vi "movetowl.vi"(8 "error out":errorcluster, 9 "GetDeviceInterface":refnum<k7>, 10 "Wavelength":dbl=795.0) -> (2 ".not. (x .or. y)?":bool)   [LabVIEW 2019]
panel:
  out "Angle":dbl
  out "Wavelength 2":dbl
  out "Serial number":string
  out "Temperature":dbl
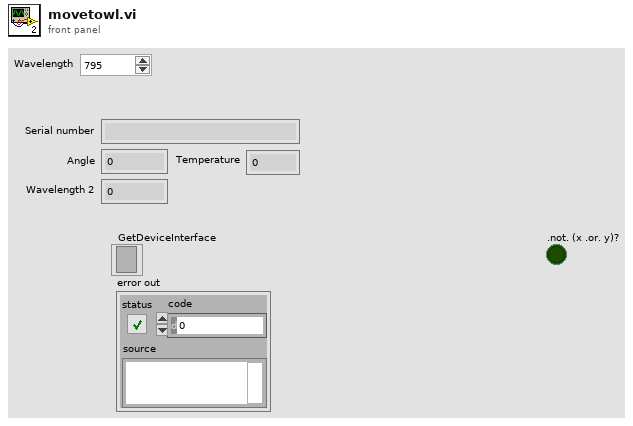
[diagram p1: front panel]
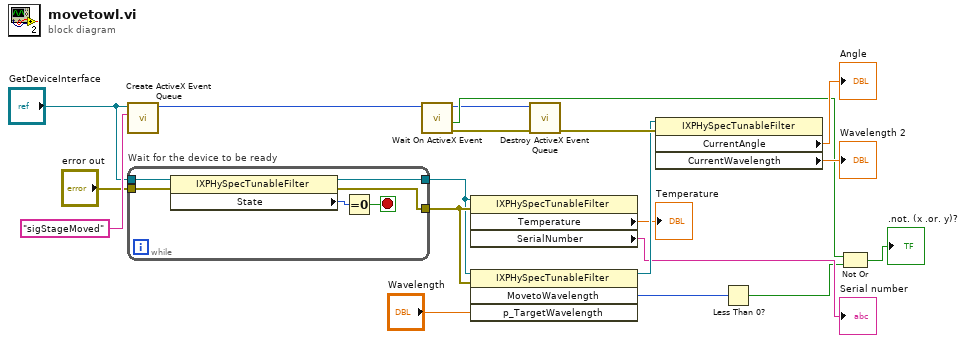
[diagram p0: block diagram]
diagram:
  n1 = call <vilib>:"Create ActiveX Event Queue.vi"("Event Name"="sigStageMoved", "Automation Refnum"="GetDeviceInterface") -> ("Event Queue"=w7:i32)  [unwired: 4 in, 1 out]
  n2 = while "Wait for the device to be ready" {
    tunnel: [w23] -> w5
    tunnel: "GetDeviceInterface" -> [w22]
    tunnel: "error out" -> [w21]
    tunnel: [w20] -> w4
    stop <- w24 stop-if-true
    n3 = property class="IXPHySpecTunableFilter"(reference=w22, error in=w21) -> (reference out=w20:refnum<k7>, error out=w23:errorcluster, "State"=w25:u32)
    n4 = Equal To 0?(x=w25) -> (x = 0?=w24:bool)
  }
  n5 = call <vilib>:"Wait On ActiveX Event.vi"("Event Queue"=w7) -> ("error out"=w9:errorcluster, "Timed Out"=w12:bool, "Event Queue Out"=w8:i32)  [unwired: 3 in, 1 out]
  n6 = property class="IXPHySpecTunableFilter"(reference=w4, error in=w5) -> ("Temperature"=→"Temperature":dbl, "SerialNumber"=→"Serial number":string)  [unwired: 2 out]
  n7 = invoke class="IXPHySpecTunableFilter" method="MovetoWavelength"(reference=w4, error in=w5, "p_TargetWavelength"="Wavelength") -> (reference out=w16:refnum<k7>, "MovetoWavelength"=w10:i32)  [unwired: 1 in, 2 out]
  n8 = call <vilib>:"Destroy ActiveX Event Queue.vi"("error in (no error)"=w9, "Event Queue"=w8) -> ("error out"=w17:errorcluster)  [unwired: 5 in]
  n9 = property class="IXPHySpecTunableFilter"(reference=w16, error in=w17) -> ("CurrentAngle"=→"Angle":dbl, "CurrentWavelength"=→"Wavelength 2":dbl)  [unwired: 2 out]
  n10 = Less Than 0?(x=w10) -> (x < 0?=w11:bool)
  n11 = Not Or(1:w11, 2:w12) -> (0:→".not. (x .or. y)?":bool)
